vi "系列号查询.vi"() -> ()   [LabVIEW 2016, in "斯坦道多参数.lvlib"]
panel:
  in  "传感器系列号":T1
  in  "布尔":bool
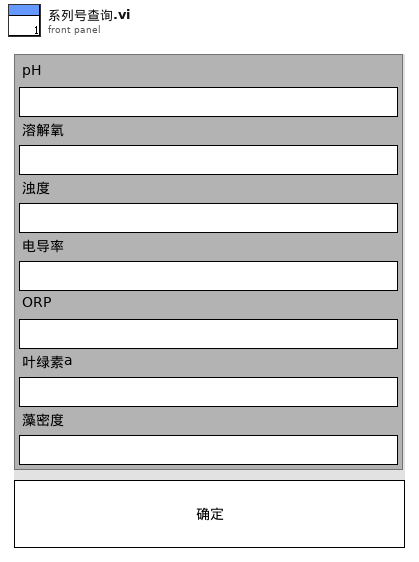
[diagram p1: front panel]
types:
  T1 = cluster{"pH":string, "溶解氧":string, "浊度":string, "电导率":string, "ORP":string, "叶绿素a":string, "藻密度":string}
  T2 = cluster{"pH探头选择":u16, "DO探头选择":u16, "电导率探头选择":u16, "浊度探头选择":u16, "叶绿素a探头选择":u16, "蓝绿藻探头选择":u16, "orp探头选择":u16, "COD探头选择":u16}
  T3 = cluster{"电极状态标志":u16, "电极型号标志":u16, "酸碱度测量值":sgl, "温度测量值":sgl, "酸碱度信号值":sgl, "温度信号值":sgl, "酸碱度偏移修正值":sgl, "温度偏移修正值":sgl, "手动温度补偿值":sgl, "酸碱度电极零点":sgl, "酸碱度电极斜率":sgl, "第1点标准值记录":sgl, "第1点信号值记录":sgl, "第1点温度值记录":sgl, "第2点标准值记录":sgl, "第2点信号值记录":sgl, "第2点温度值记录":sgl, "命令滤波设定":u16, "温度模式":enum16{"ATC", "MTC"}, "生产批次":u16, "电极序号":u16, "串口地址":u16, "串口波特率":enum16{"9600", "19200", "115200"}, "串口校验位":enum16{"NONE", "ODD", "EVEN"}, "串口停止位":enum16{"1bit", "2bit"}, "第一点标准值":sgl, "第二点标准值":sgl}
  T4 = cluster{"报警码":u16, "pH数值":sgl, "0X0003_NC":sgl, "温度数据":sgl, "pH原始信号 mv":sgl, "0X0009_NC":string, "产品名称":string, "序列号":string, "硬件版本":string, "软件版本":string, "通讯地址":u16, "波特率":u16, "设备类型":u16, "0X0026_NC":string, "第一点原始数据":sgl, "第一点校准数据":sgl, "第二点原始数据":sgl, "第二点校准数据":sgl, "探头校准命令":u16, "温度校准参数":sgl, "温度校准命令":u16}
  T5 = cluster{"电极状态标志":u16, "电极型号标志":u16, "溶解氧测量值":sgl, "温度测量值":sgl, "溶解氧饱和度值":sgl, "盐度补偿值":sgl, "大气压补偿值":sgl, "溶解氧偏移修正值":sgl, "温度偏移修正值":sgl, "手动温度补偿值":sgl, "溶解氧电极零点":sgl, "溶解氧电极斜率":sgl, "第1点标准值记录":sgl, "第1点信号值记录":sgl, "第1点温度值记录":sgl, "第2点标准值记录":sgl, "第2点信号值记录":sgl, "第2点温度值记录":sgl, "命令滤波设定":u16, "温度模式":enum16{"ATC", "MTC"}, "生产批次":u16, "电极序号":u16, "串口地址":u16, "串口波特率":enum16{"9600", "19200", "115200"}, "串口校验位":enum16{"NONE", "ODD", "EVEN"}, "串口停止位":enum16{"1bit", "2bit"}, "第一点标准值":sgl, "第二点标准值":sgl}
  T6 = cluster{"报警码":u16, "溶解氧数值（mg/L）":sgl, "溶解氧数据（%）":sgl, "温度数据":sgl, "溶解氧原始信号 nA":sgl, "大气压力":sgl, "盐度":sgl, "0X0009_NC":string, "产品名称":string, "序列号":string, "硬件版本":string, "软件版本":string, "通讯地址":u16, "波特率":u16, "设备类型":u16, "0X0026_NC":string, "第一点原始数据":sgl, "第一点校准数据":sgl, "第二点原始数据":sgl, "第二点校准数据":sgl, "探头校准命令":u16, "温度校准参数":sgl, "温度校准命令":u16}
  T7 = cluster{"电极状态标志":u16, "电极型号标志":u16, "浊度测量值":sgl, "温度测量值":sgl, "浊度信号值":sgl, "浊度偏移修正值":sgl, "温度偏移修正值":sgl, "手动温度补偿值":sgl, "浊度电极零点":sgl, "浊度电极斜率":sgl, "第1点标准值记录":sgl, "第1点信号值记录":sgl, "第1点温度值记录":sgl, "第2点标准值记录":sgl, "第2点信号值记录":sgl, "第2点温度值记录":sgl, "命令滤波设定":u16, "温度模式":enum16{"ATC", "MTC"}, "生产批次":u16, "电极序号":u16, "串口地址":u16, "串口波特率":enum16{"9600", "19200", "115200"}, "串口校验位":enum16{"NONE", "ODD", "EVEN"}, "串口停止位":enum16{"1bit", "2bit"}, "第一点标准值":sgl, "第二点标准值":sgl, "第三点标准值":sgl}
  T8 = cluster{"报警码":u16, "浊度数值 NTU":sgl, "温度数据":sgl, "原始光强数值":u16, "量程":u16, "平均次数":u16, "清扫模式":u16, "清扫次数":u16, "清扫间隔分钟":u16, "0X000B_NC":string, "产品名称":string, "序列号":string, "硬件版本":string, "软件版本":string, "通讯地址":u16, "波特率":u16, "设备类型":u16, "0X0026_NC":string, "校准量程":u16, "第一点原始光强":u16, "第一点校准数据":sgl, "第二点原始光强":u16, "第二点校准数据":sgl, "第三点原始光强":u16, "第三点校准数据":sgl, "探头校准命令":u16, "温度校准参数":sgl, "温度校准命令":u16}
  T9 = cluster{"电极状态标志":u16, "电极型号标志":u16, "电导率测量值":sgl, "温度测量值":sgl, "电导率信号值":sgl, "温度信号值":sgl, "温度补偿系数":sgl, "电导率偏移修正值":sgl, "温度偏移修正值":sgl, "手动温度补偿值":sgl, "电导率电极零点":sgl, "电导率电极斜率":sgl, "命令滤波设定":u16, "温度模式":enum16{"ATC", "MTC"}, "生产批次":u16, "电极序号":u16, "串口地址":u16, "串口波特率":enum16{"9600", "19200", "115200"}, "串口校验位":enum16{"NONE", "ODD", "EVEN"}, "串口停止位":enum16{"1bit", "2bit"}, "第一点标准值":sgl, "第二点标准值":sgl}
  T10 = cluster{"报警码":u16, "电导率数据（uS/cm）":sgl, "0x0003 NC":sgl, "温度数据":sgl, "电导率原始信号电阻":sgl, "当前量程":u16, "温度补偿系数":sgl, "0X0009_NC":string, "产品名称":string, "序列号":string, "硬件版本":string, "软件版本":string, "通讯地址":u16, "波特率":u16, "设备类型":u16, "0X0026_NC":string, "第一点原始数据":sgl, "第一点校准数据":sgl, "0X0035_NC":sgl, "0X0037_NC":sgl, "探头校准命令":u16, "温度校准参数":sgl, "温度校准命令":u16}
  T11 = cluster{"电极状态标志":u16, "电极型号标志":u16, "测量值":sgl, "温度测量值":sgl, "信号值":sgl, "温度信号值":sgl, "000AH_NC":sgl, "偏移修正值":sgl, "温度偏移修正值":sgl, "手动温度补偿值":sgl, "命令滤波设定":u16, "温度模式":enum16{"ATC", "MTC"}, "生产批次":u16, "传感器序号":u16, "串口地址":u16, "串口波特率":enum16{"9600", "19200", "115200"}, "串口校验位":enum16{"NONE", "ODD", "EVEN"}, "串口停止位":enum16{"1bit", "2bit"}}
  T12 = cluster{"报警码":u16, "叶绿素a":sgl, "温度数据":sgl, "原始光强数值":u16, "量程":u16, "平均次数":u16, "清扫模式":u16, "清扫次数":u16, "清扫间隔分钟":u16, "0X000B_NC":string, "产品名称":string, "序列号":string, "硬件版本":string, "软件版本":string, "通讯地址":u16, "波特率":u16, "设备类型":u16, "0X0026_NC":string, "校准量程":u16, "第一点原始光强":u16, "第一点校准数据":sgl, "第二点原始光强":u16, "第二点校准数据":sgl, "第三点原始光强":u16, "第三点校准数据":sgl, "探头校准命令":u16, "温度校准参数":sgl, "温度校准命令":u16}
  T13 = cluster{"报警码":u16, "蓝绿藻":sgl, "温度数据":sgl, "原始光强数值":u16, "量程":u16, "平均次数":u16, "清扫模式":u16, "清扫次数":u16, "清扫间隔分钟":u16, "0X000B_NC":string, "产品名称":string, "序列号":string, "硬件版本":string, "软件版本":string, "通讯地址":u16, "波特率":u16, "设备类型":u16, "0X0026_NC":string, "校准量程":u16, "第一点原始光强":u16, "第一点校准数据":sgl, "第二点原始光强":u16, "第二点校准数据":sgl, "第三点原始光强":u16, "第三点校准数据":sgl, "探头校准命令":u16, "温度校准参数":sgl, "温度校准命令":u16}
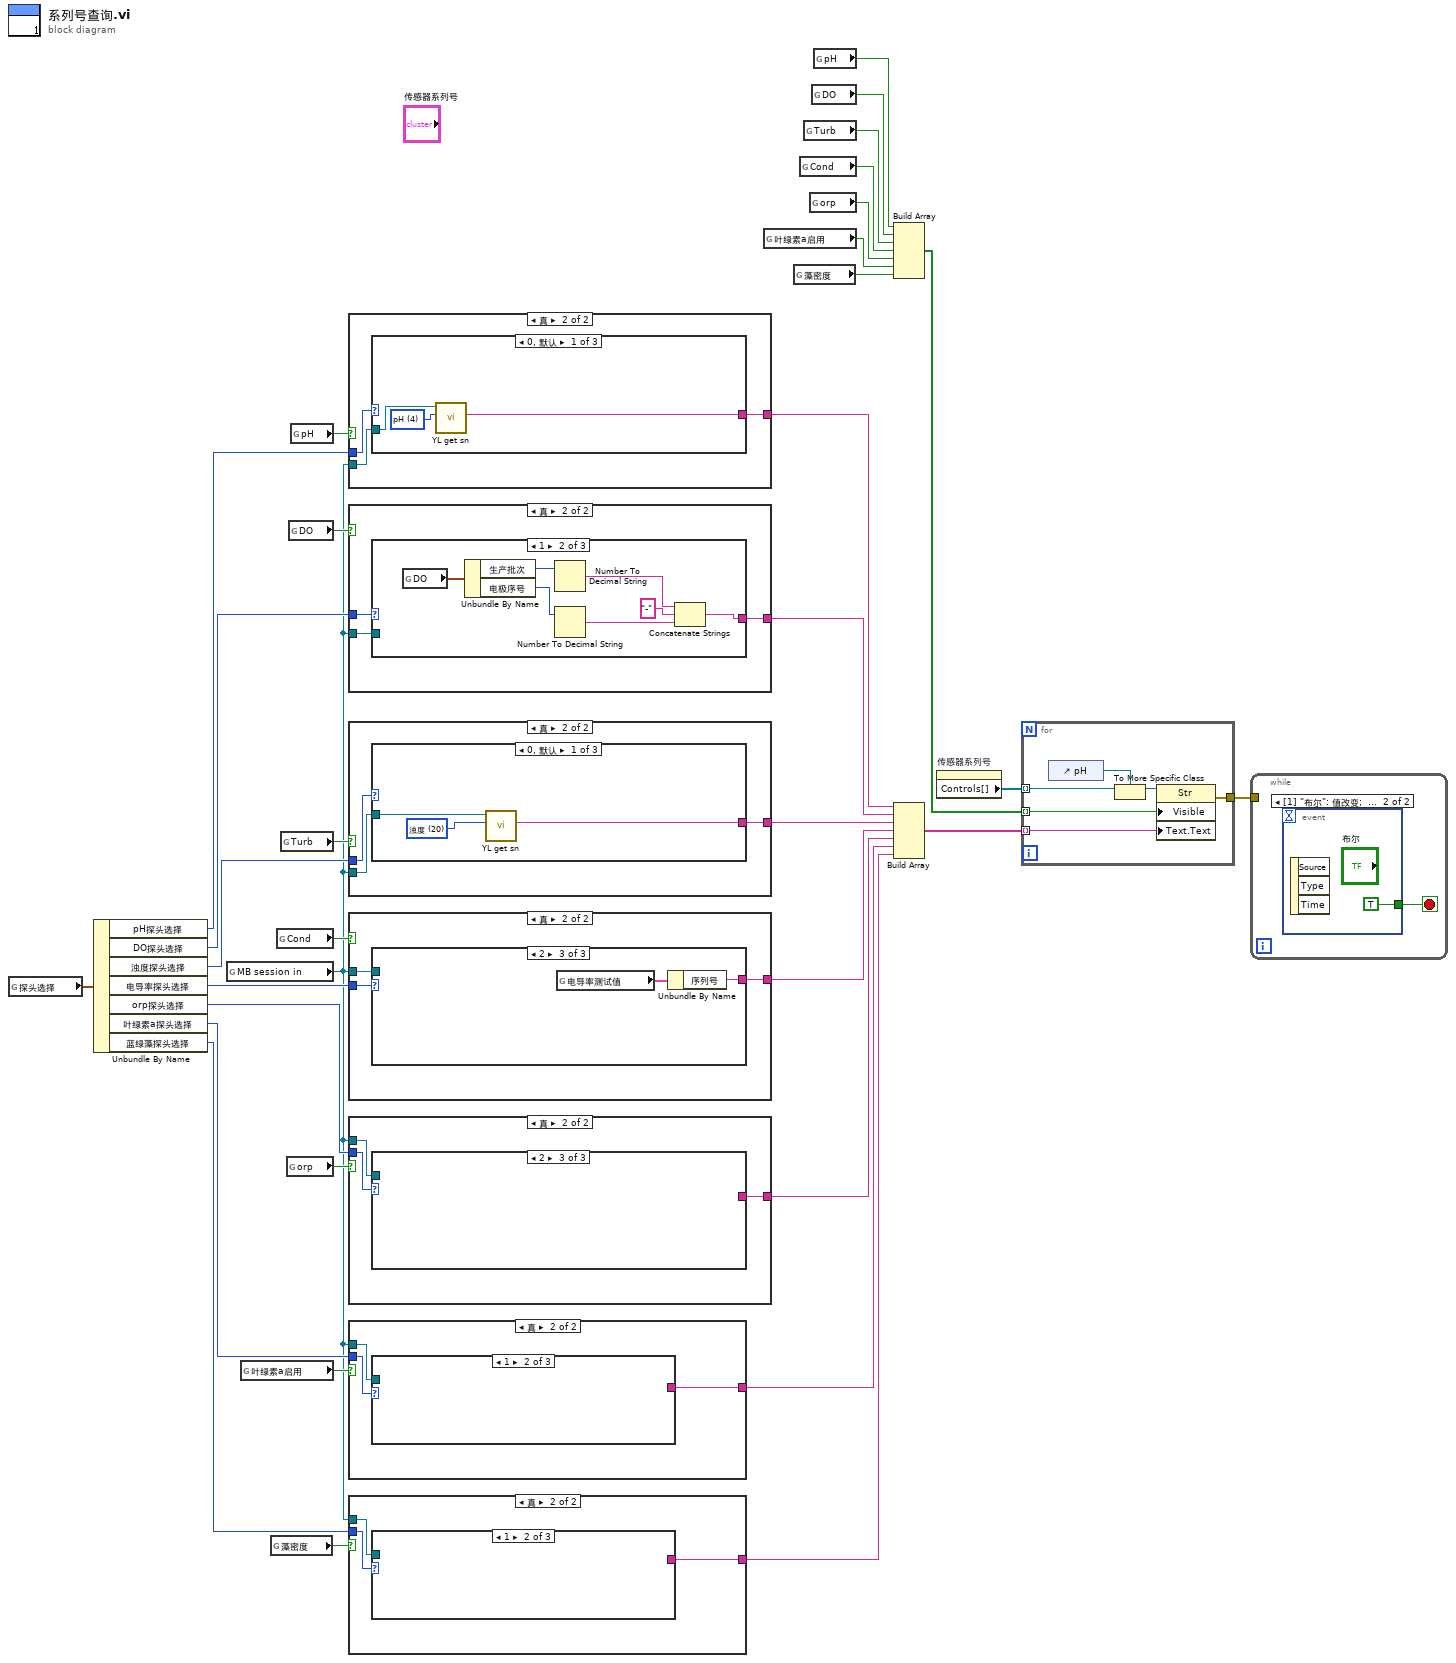
[diagram p0: block diagram]
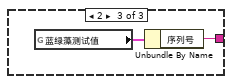
[diagram p4: hidden frame]
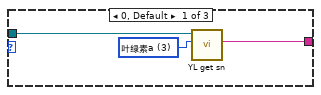
[diagram p6: hidden frame]
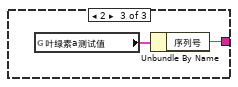
[diagram p7: hidden frame]
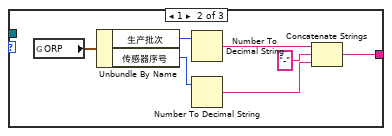
[diagram p10: hidden frame]
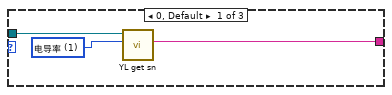
[diagram p12: hidden frame]
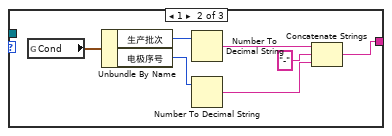
[diagram p13: hidden frame]
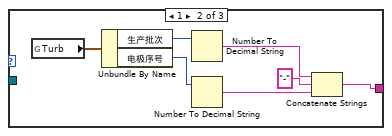
[diagram p15: hidden frame]
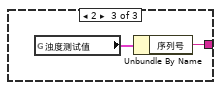
[diagram p16: hidden frame]
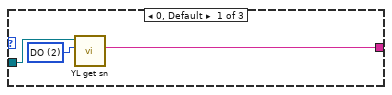
[diagram p18: hidden frame]
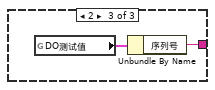
[diagram p19: hidden frame]
diagram:
  n1 = global read "断电保存变量.vi" "探头选择"() -> (w24:T2)
  n2 = Unbundle By Name(w24) -> ("pH探头选择"=w23:u16, "DO探头选择"=w21:u16, "浊度探头选择"=w19:u16, "电导率探头选择"=w16:u16, "orp探头选择"=w15:u16, "叶绿素a探头选择"=w13:u16, "蓝绿藻探头选择"=w9:u16)
  n3 = global read "多参数全局变量.vi" "MB session in"() -> (w10:refnum<class "MB_Master.lvclass">)
  n4 = global read "断电保存变量.vi" "叶绿素a启用"() -> (w12:bool)
  n5 = global read "断电保存变量.vi" "藻密度"() -> (w11:bool)
  n6 = global read "断电保存变量.vi" "Cond"() -> (w17:bool)
  n7 = global read "断电保存变量.vi" "Turb"() -> (w18:bool)
  n8 = global read "断电保存变量.vi" "orp"() -> (w14:bool)
  n9 = global read "断电保存变量.vi" "DO"() -> (w20:bool)
  n10 = global read "断电保存变量.vi" "pH"() -> (w22:bool)
  n11 = case shown="真" w22 {
    tunnel: w23 -> [_ w37]
    tunnel: [_ w36] -> w8
    tunnel: w10 -> [_ w35]
    frame False {
    }
    frame True {
      n12 = case shown="0, 默认" w37 {
        tunnel: w35 -> [w39 _ _]
        tunnel: [w38 w41 w48] -> w36
        frame 0, Default {
          w40 = u16 4 items=["电导率"=1, "DO"=2, "叶绿素a"=3, "pH"=4, "浊度"=20] ("探头型号")
          n13 = call "YL get sn.vi"("探头型号"=w40, "MB session in"=w39) -> ("SN"=w38:string)  [unwired: 7 in, 2 out]
        }
        frame 1 {
          n14 = global read "国弘过程全局变量.vi" "pH"() -> (w42:T3)
          n15 = Unbundle By Name(w42) -> ("生产批次"=w43:u16, "电极序号"=w44:u16)
          n16 = Number To Decimal String(number=w43) -> (decimal integer string=w45:string)  [unwired: 1 in]
          n17 = Number To Decimal String(number=w44) -> (decimal integer string=w46:string)  [unwired: 1 in]
          n18 = Concatenate Strings(w45, "-" ("字符串"), w46) -> (w41:string)
        }
        frame 2 {
          n19 = global read "纳清过程全局变量.vi" "pH测试值"() -> (w49:T4)
          n20 = Unbundle By Name(w49) -> ("序列号"=w48:string)
        }
      }
    }
  }
  n21 = case shown="真" w20 {
    tunnel: w21 -> [_ w52]
    tunnel: [_ w51] -> w7
    tunnel: w10 -> [_ w50]
    frame False {
    }
    frame True {
      n22 = case shown="1" w52 {
        tunnel: w50 -> [w54 _ _]
        tunnel: [w53 w56 w63] -> w51
        frame 0, Default {
          w55 = u16 2 items=["电导率"=1, "DO"=2, "叶绿素a"=3, "pH"=4, "浊度"=20] ("探头型号")
          n23 = call "YL get sn.vi"("探头型号"=w55, "MB session in"=w54) -> ("SN"=w53:string)  [unwired: 7 in, 2 out]
        }
        frame 1 {
          n24 = global read "国弘过程全局变量.vi" "DO"() -> (w57:T5)
          n25 = Unbundle By Name(w57) -> ("生产批次"=w58:u16, "电极序号"=w59:u16)
          n26 = Number To Decimal String(number=w58) -> (decimal integer string=w60:string)  [unwired: 1 in]
          n27 = Number To Decimal String(number=w59) -> (decimal integer string=w61:string)  [unwired: 1 in]
          n28 = Concatenate Strings(w60, "-" ("字符串"), w61) -> (w56:string)
        }
        frame 2 {
          n29 = global read "纳清过程全局变量.vi" "DO测试值"() -> (w64:T6)
          n30 = Unbundle By Name(w64) -> ("序列号"=w63:string)
        }
      }
    }
  }
  n31 = case shown="真" w18 {
    tunnel: w19 -> [_ w67]
    tunnel: [_ w66] -> w6
    tunnel: w10 -> [_ w65]
    frame False {
    }
    frame True {
      n32 = case shown="0, 默认" w67 {
        tunnel: w65 -> [w69 _ _]
        tunnel: [w68 w71 w78] -> w66
        frame 0, Default {
          w70 = u16 20 items=["电导率"=1, "DO"=2, "叶绿素a"=3, "pH"=4, "浊度"=20] ("探头型号")
          n33 = call "YL get sn.vi"("探头型号"=w70, "MB session in"=w69) -> ("SN"=w68:string)  [unwired: 7 in, 2 out]
        }
        frame 1 {
          n34 = global read "国弘过程全局变量.vi" "Turb"() -> (w72:T7)
          n35 = Unbundle By Name(w72) -> ("生产批次"=w73:u16, "电极序号"=w74:u16)
          n36 = Number To Decimal String(number=w73) -> (decimal integer string=w75:string)  [unwired: 1 in]
          n37 = Number To Decimal String(number=w74) -> (decimal integer string=w76:string)  [unwired: 1 in]
          n38 = Concatenate Strings(w75, "-" ("字符串"), w76) -> (w71:string)
        }
        frame 2 {
          n39 = global read "纳清过程全局变量.vi" "浊度测试值"() -> (w79:T8)
          n40 = Unbundle By Name(w79) -> ("序列号"=w78:string)
        }
      }
    }
  }
  n41 = case shown="真" w17 {
    tunnel: w16 -> [_ w82]
    tunnel: [_ w81] -> w5
    tunnel: w10 -> [_ w80]
    frame False {
    }
    frame True {
      n42 = case shown="2" w82 {
        tunnel: w80 -> [w84 _ _]
        tunnel: [w83 w86 w93] -> w81
        frame 0, Default {
          w85 = u16 1 items=["电导率"=1, "DO"=2, "叶绿素a"=3, "pH"=4, "浊度"=20] ("探头型号")
          n43 = call "YL get sn.vi"("探头型号"=w85, "MB session in"=w84) -> ("SN"=w83:string)  [unwired: 7 in, 2 out]
        }
        frame 1 {
          n44 = global read "国弘过程全局变量.vi" "Cond"() -> (w87:T9)
          n45 = Unbundle By Name(w87) -> ("生产批次"=w88:u16, "电极序号"=w89:u16)
          n46 = Number To Decimal String(number=w88) -> (decimal integer string=w90:string)  [unwired: 1 in]
          n47 = Number To Decimal String(number=w89) -> (decimal integer string=w91:string)  [unwired: 1 in]
          n48 = Concatenate Strings(w90, "-" ("字符串"), w91) -> (w86:string)
        }
        frame 2 {
          n49 = global read "纳清过程全局变量.vi" "电导率测试值"() -> (w94:T10)
          n50 = Unbundle By Name(w94) -> ("序列号"=w93:string)
        }
      }
    }
  }
  n51 = case shown="真" w14 {
    tunnel: w15 -> [_ w97]
    tunnel: [_ w96] -> w4
    tunnel: w10 -> [_ w95]
    frame False {
    }
    frame True {
      n52 = case shown="2" w97 {
        tunnel: w95 -> [_ _ _]
        tunnel: [_ w98 _] -> w96
        frame 0, Default {
        }
        frame 1 {
          n53 = global read "国弘过程全局变量.vi" "ORP"() -> (w99:T11)
          n54 = Unbundle By Name(w99) -> ("生产批次"=w100:u16, "传感器序号"=w101:u16)
          n55 = Number To Decimal String(number=w100) -> (decimal integer string=w102:string)  [unwired: 1 in]
          n56 = Number To Decimal String(number=w101) -> (decimal integer string=w103:string)  [unwired: 1 in]
          n57 = Concatenate Strings(w102, "-" ("字符串"), w103) -> (w98:string)
        }
        frame 2 {
        }
      }
    }
  }
  n58 = case shown="真" w12 {
    tunnel: w13 -> [_ w107]
    tunnel: [_ w106] -> w3
    tunnel: w10 -> [_ w105]
    frame False {
    }
    frame True {
      n59 = case shown="1" w107 {
        tunnel: w105 -> [w109 _ _]
        tunnel: [w108 _ w111] -> w106
        frame 0, Default {
          w110 = u16 3 items=["电导率"=1, "DO"=2, "叶绿素a"=3, "pH"=4, "浊度"=20] ("探头型号")
          n60 = call "YL get sn.vi"("探头型号"=w110, "MB session in"=w109) -> ("SN"=w108:string)  [unwired: 7 in, 2 out]
        }
        frame 1 {
        }
        frame 2 {
          n61 = global read "纳清过程全局变量.vi" "叶绿素a测试值"() -> (w112:T12)
          n62 = Unbundle By Name(w112) -> ("序列号"=w111:string)
        }
      }
    }
  }
  n63 = case shown="真" w11 {
    tunnel: w9 -> [_ w115]
    tunnel: [_ w114] -> w2
    tunnel: w10 -> [_ w113]
    frame False {
    }
    frame True {
      n64 = case shown="1" w115 {
        tunnel: w113 -> [_ _ _]
        tunnel: [_ _ w116] -> w114
        frame 0, Default {
        }
        frame 1 {
        }
        frame 2 {
          n65 = global read "纳清过程全局变量.vi" "蓝绿藻测试值"() -> (w117:T13)
          n66 = Unbundle By Name(w117) -> ("序列号"=w116:string)
        }
      }
    }
  }
  n67 = global read "断电保存变量.vi" "叶绿素a启用"() -> (w29:bool)
  n68 = global read "断电保存变量.vi" "藻密度"() -> (w28:bool)
  n69 = global read "断电保存变量.vi" "Cond"() -> (w31:bool)
  n70 = global read "断电保存变量.vi" "Turb"() -> (w32:bool)
  n71 = global read "断电保存变量.vi" "orp"() -> (w30:bool)
  n72 = global read "断电保存变量.vi" "DO"() -> (w33:bool)
  n73 = global read "断电保存变量.vi" "pH"() -> (w34:bool)
  n74 = Build Array(w34, w33, w32, w31, w30, w29, w28) -> (w26:bool[])
  n75 = Build Array(w8, w7, w6, w5, w4, w3, w2) -> (w1:string[])
  n76 = property on="传感器系列号" class="Clust (严格)"() -> ("Controls[]"=w27:refnum<vi>[])  [unwired: 2 in, 2 out]
  n77 = for {
    tunnel: w27 -> [w121] mode=indexing
    tunnel: w26 -> [w123] mode=indexing
    tunnel: [w122] -> w25
    tunnel: w1 -> [w118] mode=indexing
    n78 = control-ref of="pH"() -> (w120:refnum<vi>)
    n79 = To More Specific Class(target class=w120, reference=w121) -> (specific class reference=w119:refnum<vi>)  [unwired: 1 in, 1 out]
    n80 = property class="Str"(reference=w119, "Visible"=w123, "Text.Text"=w118) -> (error out=w122:errorcluster)  [unwired: 1 in, 1 out]
  }
  n81 = while {
    tunnel: w25 -> [_]
    stop <- w124 stop-if-true
    n82 = event shown="[1] \"布尔\": 值改变;  前面板关闭" {
      selector: _ -> [_ _]
      dyn-events: _ -> [_ _]
      timeout: _ -> [_ _]
      tunnel: [_ TRUE] -> w124
      event Timeout {
        n83 = event-data() -> ()  [unwired: 1 in, 3 out]
      }
      event "布尔": Value Change; Panel Close {
        n84 = event-data() -> ()  [unwired: 1 in, 3 out]
      }
    }
  }
